vi "PYBD-OpenMV.vi"() -> ()   [LabVIEW 2016]
uses:
  VIs/uPythonX/uPythonX.xctl
panel:
  in  "stop":bool
  out "Console Out 2":string="\r\n>>> import os\r\n>>> \r\n>>> file = open('main.py','wb')\r\n>>> text = file.write(b'\\x69\\x6D\\x70\\x6F\\x72\\x74\\x20\\x6D\\x61\\x63\\x68\\x69\\x6E\\x65\\x2C\\x20\\x75\\x74\\x69\\x6D\\x65\\x0A\\x0A\\x66\\x72\\x6F\\x6D\\x20\\x70\\x79\\x62\\x20\\x69\\x6D\\x70\\x6F\\x72\\x74\\x20\\x4C\\x45\\x44\\x0A\\x0A\\x23\\x20\\x52\\x65\\x61\\x64\\x20\\x28\\x31\\x29\\x20\\x47\\x72\\x65\\x65\\x6E\\x20\\x28\\x32\\x29\\x20\\x59\\x65\\x6C\\x6C\\x6F\\x77\\x20\\x28\\x33\\x29\\x20\\x61\\x6E\\x64\\x20\\x42\\x6C\\x75\\x65\\x20\\x28\\x34\\x29\\x0A\\x0A\\x6C\\x65\\x64\\x20\\x3D\\x20\\x4C\\x45\\x44\\x28\\x31\\x29\\x0A\\x0A\\x75\\x61\\x72\\x74\\x20\\x3D\\x20\\x6D\\x61\\x63\\x68\\x69\\x6E\\x65\\x2E\\x55\\x41\\x52\\x54\\x28\\x33\\x29\\x0A\\x75\\x61\\x72\\x74\\x2E\\x69\\x6E\\x69\\x74\\x28\\x62\\x61\\x75\\x64\\x72\\x61\\x74\\x65\\x3D\\x32\\x34\\x30\\x30\\x2C\\x20\\x62\\x69\\x74\\x73\\x3D\\x38\\x2C\\x20\\x70\\x61\\x72\\x69\\x74\\x79\\x3D\\x4E\\x6F\\x6E\\x65\\x2C\\x20\\x73\\x74\\x6F\\x70\\x3D\\x31\\x29\\x0A\\x0A\\x77\\x68\\x69\\x6C\\x65\\x20\\x54\\x72\\x75\\x65\\x3A\\x0A\\x20\\x20\\x20\\x20\\x20\\x75\\x61\\x72\\x74\\x2E\\x77\\x72\\x69\\x74\\x65\\x28\\x62\\x27\\x5C\\x5C\\x78\\x32\\x32\\x27\\x29\\x0A\\x20\\x20\\x20\\x20\\x20\\x73\\x69\\x7A\\x65\\x20\\x3D\\x20\\x75\\x61\\x72\\x74\\x2E\\x61\\x6E\\x79\\x28\\x29\\x0A\\x20\\x20\\x20\\x20\\x20\\x70\\x72\\x69\\x6E\\x74\\x28\\x75\\x61\\x72\\x74\\x2E\\x72\\x65\\x61\\x64\\x28\\x73\\x69\\x7A\\x65\\x29\\x29\\x0A\\x20\\x20\\x20\\x20\\x20\\x75\\x74\\x69\\x6D\\x65\\x2E\\x73\\x6C\\x65\\x65\\x70\\x28\\x31\\x29\\x0A\\x20\\x20\\x20\\x20\\x20\\x6C\\x65\\x64\\x2E\\x74\\x6F\\x67\\x67\\x6C\\x65\\x28\\x29\\x0A')\r\n>>> file.close()\r\n>>> text\r\n309\r\n>>> \r\nMicroPython v1.9.4-4531-g65b367440 on 2018-11-04; OPENMV3 with STM32F765\r\nType \"help()\" for more information.\r\n>>> "
  out "Console Out":string="MicroPython v1.10-212-g8fa343f6e-dirty on 2019-02-03; PYBD_SF2 with STM32F722IEK\r\nType \"help()\" for more information.\r\n>>> \r\n>>> import os\r\n>>> \r\n>>> file = open('main.py','wb')\r\n>>> text = file.write(b'\\x69\\x6D\\x70\\x6F\\x72\\x74\\x20\\x6D\\x61\\x63\\x68\\x69\\x6E\\x65\\x2C\\x20\\x75\\x74\\x69\\x6D\\x65\\x0A\\x0A\\x66\\x72\\x6F\\x6D\\x20\\x70\\x79\\x62\\x20\\x69\\x6D\\x70\\x6F\\x72\\x74\\x20\\x4C\\x45\\x44\\x0A\\x0A\\x23\\x20\\x52\\x65\\x61\\x64\\x20\\x28\\x31\\x29\\x20\\x47\\x72\\x65\\x65\\x6E\\x20\\x28\\x32\\x29\\x20\\x59\\x65\\x6C\\x6C\\x6F\\x77\\x20\\x28\\x33\\x29\\x20\\x61\\x6E\\x64\\x20\\x42\\x6C\\x75\\x65\\x20\\x28\\x34\\x29\\x0A\\x0A\\x6C\\x65\\x64\\x20\\x3D\\x20\\x4C\\x45\\x44\\x28\\x31\\x29\\x0A\\x0A\\x75\\x61\\x72\\x74\\x20\\x3D\\x20\\x6D\\x61\\x63\\x68\\x69\\x6E\\x65\\x2E\\x55\\x41\\x52\\x54\\x28\\x33\\x29\\x0A\\x75\\x61\\x72\\x74\\x2E\\x69\\x6E\\x69\\x74\\x28\\x62\\x61\\x75\\x64\\x72\\x61\\x74\\x65\\x3D\\x32\\x34\\x30\\x30\\x2C\\x20\\x62\\x69\\x74\\x73\\x3D\\x38\\x2C\\x20\\x70\\x61\\x72\\x69\\x74\\x79\\x3D\\x4E\\x6F\\x6E\\x65\\x2C\\x20\\x73\\x74\\x6F\\x70\\x3D\\x31\\x29\\x0A\\x0A\\x77\\x68\\x69\\x6C\\x65\\x20\\x54\\x72\\x75\\x65\\x3A\\x0A\\x20\\x20\\x20\\x20\\x20\\x75\\x61\\x72\\x74\\x2E\\x77\\x72\\x69\\x74\\x65\\x28\\x62\\x27\\x5C\\x5C\\x78\\x32\\x32\\x27\\x29\\x0A\\x20\\x20\\x20\\x20\\x20\\x73\\x69\\x7A\\x65\\x20\\x3D\\x20\\x75\\x61\\x72\\x74\\x2E\\x61\\x6E\\x79\\x28\\x29\\x0A\\x20\\x20\\x20\\x20\\x20\\x70\\x72\\x69\\x6E\\x74\\x28\\x75\\x61\\x72\\x74\\x2E\\x72\\x65\\x61\\x64\\x28\\x73\\x69\\x7A\\x65\\x29\\x29\\x0A\\x20\\x20\\x20\\x20\\x20\\x75\\x74\\x69\\x6D\\x65\\x2E\\x73\\x6C\\x65\\x65\\x70\\x28\\x31\\x29\\x0A\\x20\\x20\\x20\\x20\\x20\\x6C\\x65\\x64\\x2E\\x74\\x6F\\x67\\x67\\x6C\\x65\\x28\\x29\\x0A')\r\n>>> file.close()\r\n>>> text\r\n309\r\n>>> \r\nPYB: sync filesystems\r\nPYB: soft reboot\r\nb''\r\nb''\r\nb''\r\nb''\r\n"
  in  "OpenMV":T1(xcontrol)={"VISA Refnum in"="ASRL12::INSTR", "Python Code"="import machine, utime\n\nfrom pyb import LED\n\n# Read (1) Green (2) Yellow (3) and Blue (4)\n\nled = LED(1)\n\nuart = machine.UART(3)\nuart.init(baudrate=2400, bits=8, parity=None, stop=1)\n\nwhile True:\n     uart.write(b'\\\\x22')\n     size = uart.any()\n     print(uart.read(size))\n     utime.sleep(1)\n     led.toggle()\n"}
  in  "PYBD":T1(xcontrol)={"VISA Refnum in"="ASRL32::INSTR", "Python Code"="import machine, utime\n\nfrom pyb import LED\n\n# Read (1) Green (2) Yellow (3) and Blue (4)\n\nled = LED(1)\n\nuart = machine.UART(3)\nuart.init(baudrate=2400, bits=8, parity=None, stop=1)\n\nwhile True:\n     uart.write(b'\\\\x22')\n     size = uart.any()\n     print(uart.read(size))\n     utime.sleep(1)\n     led.toggle()\n"}
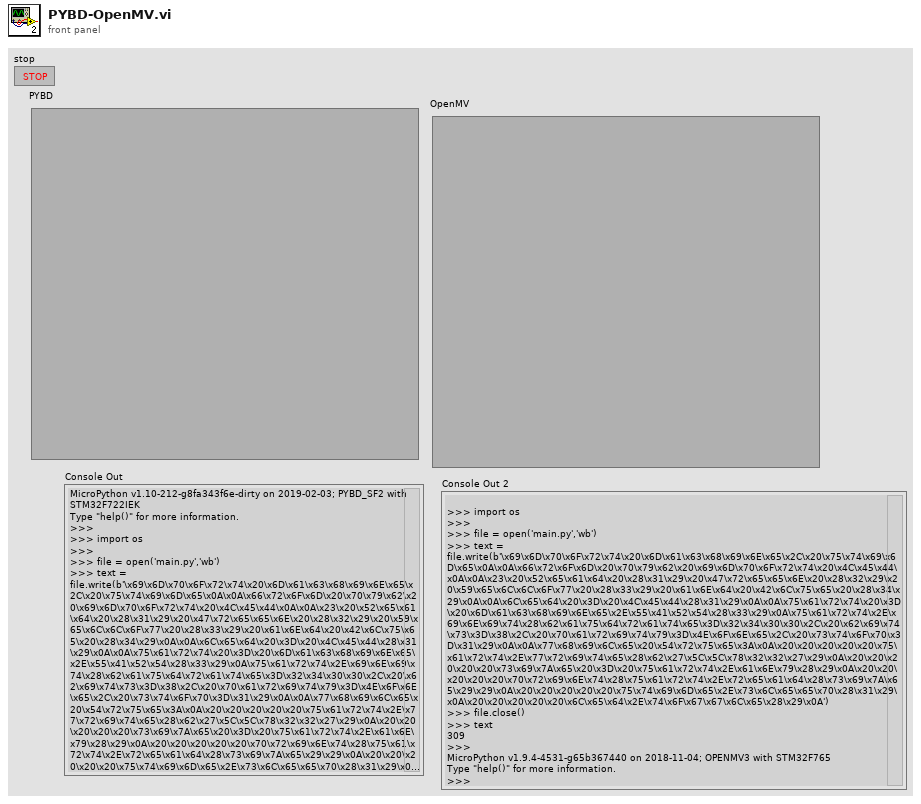
[diagram p1: front panel]
types:
  T1 = cluster{"VISA Refnum in":refnum<visa-resource-name>, "Python Code":string}
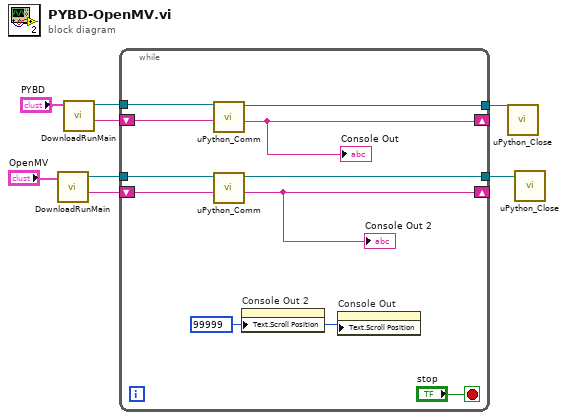
[diagram p0: block diagram]
diagram:
  n1 = call "DownloadRunMain.vi"("uPythonX"="OpenMV") -> ("Reply"=w4:string, "VISA Refnum out"=w5:refnum<visa-resource-name>)  [unwired: 8 in, 1 out]
  n2 = call "DownloadRunMain.vi"("uPythonX"="PYBD") -> ("Reply"=w3:string, "VISA Refnum out"=w6:refnum<visa-resource-name>)  [unwired: 8 in, 1 out]
  n3 = while {
    tunnel: w6 -> [w18]
    tunnel: w5 -> [w17]
    shift-right: [w15] -> _
    shift-left: w4 -> [w16]
    shift-right: [w13] -> _
    shift-left: w3 -> [w14]
    tunnel: [w11] -> w2
    tunnel: [w10] -> w1
    stop <- "stop" stop-if-true
    w9 = u32 99999 ("Text.Scroll Position")
    n4 = call "uPython_Comm.vi"("Console In"=w14, "VISA Refnum in"=w18) -> ("Console Out"=w13:string, "VISA out"=w10:refnum<visa-resource-name>)  [unwired: 5 in, 3 out]
    "Console Out" <- w13
    n5 = call "uPython_Comm.vi"("Console In"=w16, "VISA Refnum in"=w17) -> ("Console Out"=w15:string, "VISA out"=w11:refnum<visa-resource-name>)  [unwired: 5 in, 3 out]
    "Console Out 2" <- w15
    n6 = property on="Console Out 2" class="Str"("Text.Scroll Position"=w9) -> ()  [unwired: 2 in, 2 out]
    n7 = property on="Console Out" class="Str"("Text.Scroll Position"=w9) -> ()  [unwired: 2 in, 2 out]
  }
  n8 = call "uPython_Close.vi"("VISA  in"=w1) -> ()  [unwired: 9 in, 2 out]
  n9 = call "uPython_Close.vi"("VISA  in"=w2) -> ()  [unwired: 9 in, 2 out]
